vi "saveNodes.vi"(6 "Save As":bool, 8 "error in (no error)":errorcluster, 11 "xceRootNode in":refnum<class "xceRootNode.lvclass">) -> (0 "error out":errorcluster, 1 "cancelled":bool, 3 "xceRootNode out":refnum<class "xceRootNode.lvclass">)   [LabVIEW 2013, in "xceRootNode.lvclass"]
doc: "Saves the tree data structure to file without a prompt."
uses:
  xceRootNode.lvclass
  xceRootNode.lvclass/xceRootNode.ctl
  xceDataNode/xceDataNode.lvclass
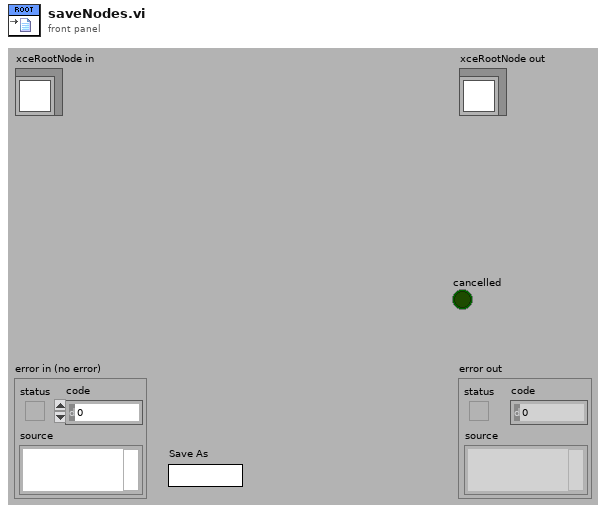
[diagram p1: front panel]
types:
  T1 = enum16{"open", "replace", "create", "open or create", "replace or create", "replace or create with confirmation"}
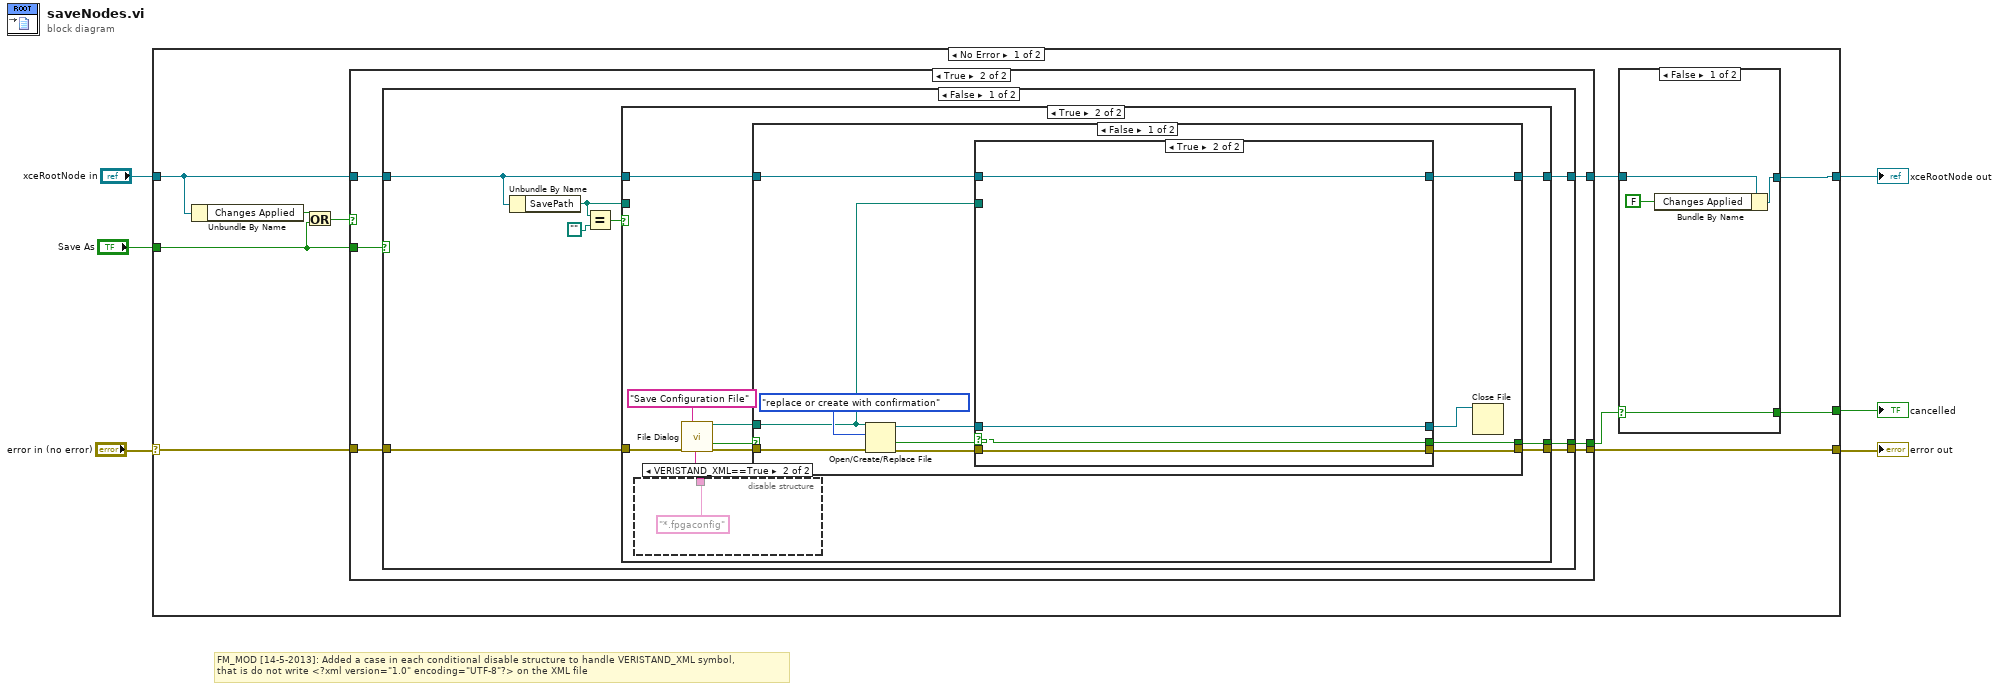
[diagram p0: block diagram]
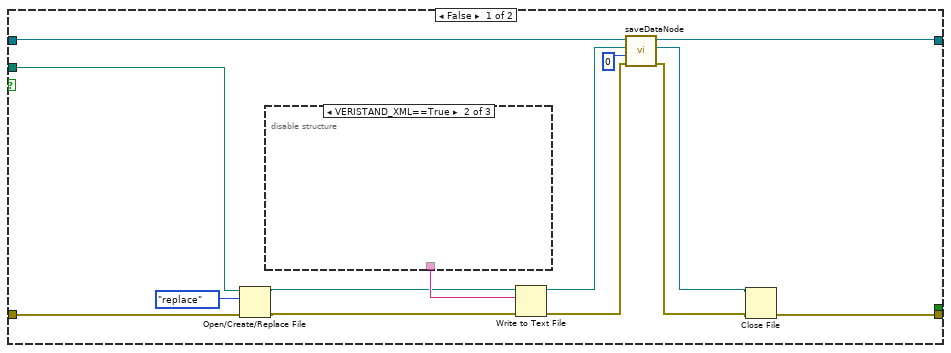
[diagram p4: hidden frame]
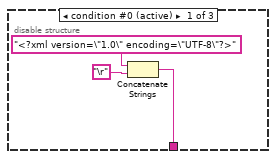
[diagram p5: hidden frame]
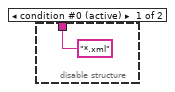
[diagram p7: hidden frame]
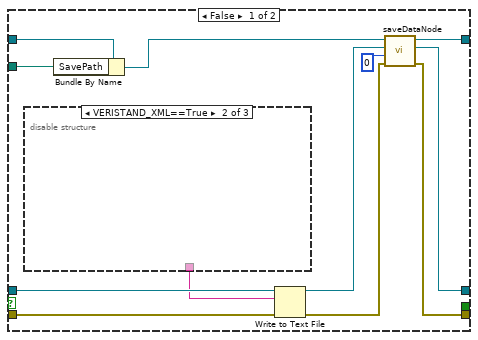
[diagram p8: hidden frame]
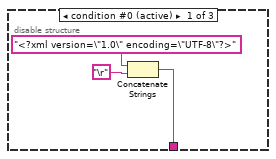
[diagram p9: hidden frame]
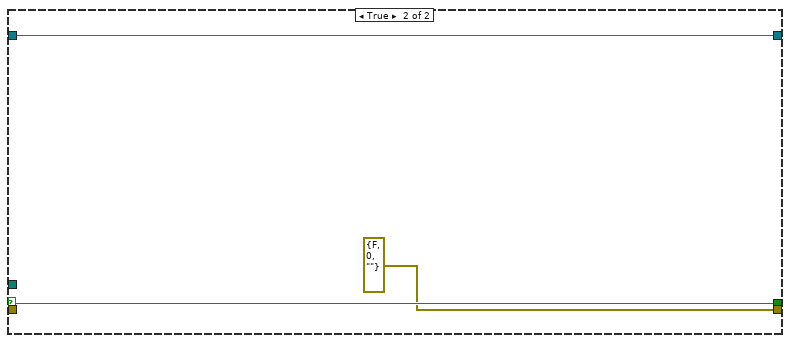
[diagram p11: hidden frame]
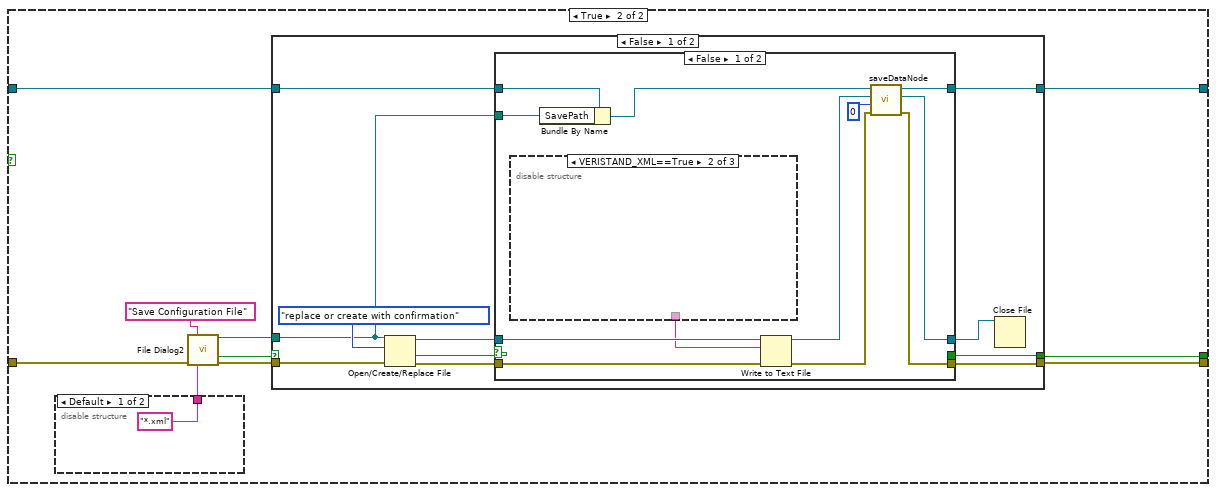
[diagram p12: hidden frame]
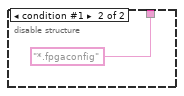
[diagram p13: hidden frame]
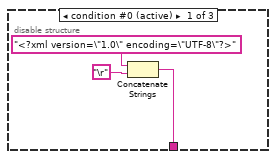
[diagram p14: hidden frame]
diagram:
  # "FM_MOD [14-5-2013]: Added a case in each conditional disable structure to handle VERISTAND_XML symbol,\nthat is do not write <?xml version=\"1.0\" encoding=\"UTF-8\"?> on the XML file"
  n1 = case shown="No Error" "error in (no error)" {
    selector: "error in (no error)" -> [w15 w147]
    tunnel: [w12 w147] -> w5
    tunnel: [w7 w146] -> w3
    tunnel: "xceRootNode in" -> [w13 w146]
    tunnel: "Save As" -> [w11 _]
    tunnel: [w9 _] -> w1
    frame No Error {
      n2 = Unbundle By Name(w13) -> ("Changes Applied"=w16:bool)
      n3 = Or(x=w16, y=w11) -> (x .or. y?=w14:bool)
      n4 = case shown="True" w14 {
        tunnel: w15 -> [w24 w28]
        tunnel: w13 -> [w23 w29]
        tunnel: [w23 w27] -> w8
        tunnel: [w24 w25] -> w12
        tunnel: w11 -> [_ w30]
        tunnel: [_ w26] -> w10
        frame False {
        }
        frame True {
          n5 = case shown="False" w30 {
            tunnel: w29 -> [w35 w105]
            tunnel: w28 -> [w36 w104]
            tunnel: [w34 w101] -> w27
            tunnel: [w33 w102] -> w26
            tunnel: [w32 w103] -> w25
            frame False {
              n6 = Unbundle By Name(w35) -> ("SavePath"=w31:path)
              n7 = Equal?(x=w31, y=path "") -> (x = y?=w37:bool)
              n8 = case shown="True" w37 {
                tunnel: w36 -> [w52 w64]
                tunnel: w35 -> [w45 w60]
                tunnel: [w44 w59] -> w34
                tunnel: [_ w58] -> w33
                tunnel: [w41 w57] -> w32
                tunnel: w31 -> [w51 _]
                frame False {
                  n9 = Open/Create/Replace File(file path (use dialog)=w51, error in=w52, operation (0:open)=T1."replace") -> (refnum out=w40:refnum<file>, error out=w39:errorcluster)  [unwired: 3 in, 1 out]
                  n10 = disable-structure shown="VERISTAND_XML==True" {
                    disable-tunnel: [w53 _ _] -> w49
                    frame condition #0 (active) {
                      n11 = Concatenate Strings("<?xml version=\"1.0\" encoding=\"UTF-8\"?>", "\r") -> (w53:string)
                    }
                    frame condition #1 {
                    }
                    frame condition #2 {
                    }
                  }
                  n12 = Write to Text File(file (use dialog)=w40, text=w49, error in=w39) -> (refnum out=w47:refnum<file>, error out=w48:errorcluster)  [unwired: 1 in, 1 out]
                  n13 = call "saveDataNode.vi"("error in (no error)"=w48, "indent"=0, "XML Refnum in"=w47, "xceDataNode in"=w45) -> ("error out"=w42:errorcluster, "XML Refnum out"=w43:refnum<file>, "xceDataNode out"=w44:refnum<class "xceRootNode.lvclass">)  [unwired: 5 in]
                  n14 = Close File(refnum=w43, error in=w42) -> (error out=w41:errorcluster)  [unwired: 1 out]
                }
                frame True {
                  n15 = disable-structure shown="VERISTAND_XML==True" {
                    disable-tunnel: ["*.xml" ("pattern (all files)") "*.fpgaconfig" ("pattern (all files)")] -> w56
                    frame condition #0 (active) {
                    }
                    frame condition #1 {
                    }
                  }
                  n16 = call "File Dialog"("prompt"="Save Configuration File", "error in"=w64, "pattern (all files)"=w56) -> ("selected path"=w61:path, "cancelled"=w63:bool, "error out"=w62:errorcluster)  [unwired: 9 in, 1 out]
                  n17 = case shown="False" w63 {
                    selector: w63 -> [_ w99]
                    tunnel: w62 -> [w77 _]
                    tunnel: w61 -> [w68 _]
                    tunnel: w60 -> [w70 w100]
                    tunnel: [w69 w100] -> w59
                    tunnel: [w75 w99] -> w58
                    tunnel: [w72 errorcluster {"status"=FALSE, "code"=0, "source"=""} ("error out")] -> w57
                    frame False {
                      n18 = Open/Create/Replace File(file path (use dialog)=w68, error in=w77, operation (0:open)=T1."replace or create with confirmation") -> (refnum out=w73:refnum<file>, cancelled=w74:bool, error out=w76:errorcluster)  [unwired: 3 in]
                      n19 = case shown="True" w74 {
                        selector: w74 -> [_ w96]
                        tunnel: w76 -> [w88 w97]
                        tunnel: [w85 w97] -> w72
                        tunnel: [_ w96] -> w75
                        tunnel: w73 -> [w90 w95]
                        tunnel: [w84 w95] -> w71
                        tunnel: w70 -> [w80 w94]
                        tunnel: [w87 w94] -> w69
                        tunnel: w68 -> [w81 _]
                        frame False {
                          n20 = disable-structure shown="VERISTAND_XML==True" {
                            disable-tunnel: [w91 _ _] -> w89
                            frame condition #0 (active) {
                              n21 = Concatenate Strings("<?xml version=\"1.0\" encoding=\"UTF-8\"?>", "\r") -> (w91:string)
                            }
                            frame condition #1 {
                            }
                            frame condition #2 {
                            }
                          }
                          n22 = Bundle By Name(cluster=w80, "SavePath"=w81) -> (w79:refnum<class "xceRootNode.lvclass">)
                          n23 = Write to Text File(file (use dialog)=w90, text=w89, error in=w88) -> (refnum out=w83:refnum<file>, error out=w86:errorcluster)  [unwired: 1 in, 1 out]
                          n24 = call "saveDataNode.vi"("error in (no error)"=w86, "indent"=0, "XML Refnum in"=w83, "xceDataNode in"=w79) -> ("error out"=w85:errorcluster, "XML Refnum out"=w84:refnum<file>, "xceDataNode out"=w87:refnum<class "xceRootNode.lvclass">)  [unwired: 5 in]
                        }
                        frame True {
                        }
                      }
                      n25 = Close File(refnum=w71) -> ()  [unwired: 1 in, 2 out]
                    }
                    frame True {
                    }
                  }
                }
              }
            }
            frame True {
              n26 = disable-structure shown="Default" {
                disable-tunnel: ["*.xml" ("pattern (all files)") "*.fpgaconfig" ("pattern (all files)")] -> w110
                frame condition #0 (active) {
                }
                frame condition #1 {
                }
              }
              n27 = call "File Dialog2"("prompt"="Save Configuration File", "error in"=w104, "pattern (all files)"=w110) -> ("selected path"=w106:path, "cancelled"=w108:bool, "error out"=w107:errorcluster)  [unwired: 9 in, 1 out]
              n28 = case shown="False" w108 {
                selector: w108 -> [_ w144]
                tunnel: w107 -> [w122 w143]
                tunnel: w106 -> [w113 _]
                tunnel: w105 -> [w115 w145]
                tunnel: [w114 w145] -> w101
                tunnel: [w120 w144] -> w102
                tunnel: [w117 w143] -> w103
                frame False {
                  n29 = Open/Create/Replace File(file path (use dialog)=w113, error in=w122, operation (0:open)=T1."replace or create with confirmation") -> (refnum out=w118:refnum<file>, cancelled=w119:bool, error out=w121:errorcluster)  [unwired: 3 in]
                  n30 = case shown="False" w119 {
                    selector: w119 -> [_ w141]
                    tunnel: w121 -> [w133 w142]
                    tunnel: [w130 w142] -> w117
                    tunnel: [_ w141] -> w120
                    tunnel: w118 -> [w135 w140]
                    tunnel: [w129 w140] -> w116
                    tunnel: w115 -> [w125 w139]
                    tunnel: [w132 w139] -> w114
                    tunnel: w113 -> [w126 _]
                    frame False {
                      n31 = disable-structure shown="VERISTAND_XML==True" {
                        disable-tunnel: [w136 _ _] -> w134
                        frame condition #0 (active) {
                          n32 = Concatenate Strings("<?xml version=\"1.0\" encoding=\"UTF-8\"?>", "\r") -> (w136:string)
                        }
                        frame condition #1 {
                        }
                        frame condition #2 {
                        }
                      }
                      n33 = Bundle By Name(cluster=w125, "SavePath"=w126) -> (w124:refnum<class "xceRootNode.lvclass">)
                      n34 = Write to Text File(file (use dialog)=w135, text=w134, error in=w133) -> (refnum out=w128:refnum<file>, error out=w131:errorcluster)  [unwired: 1 in, 1 out]
                      n35 = call "saveDataNode.vi"("error in (no error)"=w131, "indent"=0, "XML Refnum in"=w128, "xceDataNode in"=w124) -> ("error out"=w130:errorcluster, "XML Refnum out"=w129:refnum<file>, "xceDataNode out"=w132:refnum<class "xceRootNode.lvclass">)  [unwired: 5 in]
                    }
                    frame True {
                    }
                  }
                  n36 = Close File(refnum=w116) -> ()  [unwired: 1 in, 2 out]
                }
                frame True {
                }
              }
            }
          }
        }
      }
      n37 = case shown="False" w10 {
        selector: w10 -> [w20 w21]
        tunnel: [w20 w21] -> w9
        tunnel: w8 -> [w19 w22]
        tunnel: [w17 w22] -> w7
        frame False {
          n38 = Bundle By Name(cluster=w19, "Changes Applied"=FALSE) -> (w17:refnum<class "xceRootNode.lvclass">)
        }
        frame True {
        }
      }
    }
    frame Error {
    }
  }
  "error out" <- w5
  "xceRootNode out" <- w3
  "cancelled" <- w1
